vi "Drive_Motion_Control.vi"() -> ()   [LabVIEW 2017]
uses:
  State Control.ctl
panel:
  in  "Emergency Stop":bool
  out "Position":dbl(graph)
  out "Velocity":dbl(graph)
  in  "Move Absolute":bool
  in  "Move to Absolute Position in inches":dbl=1.0 min=1.0 max=20.0
  out "Motion in progress":bool
  in  "Homing":bool
  out "Sending in Progress":bool
  in  "Quit":bool
  in  "Motion Relative to Current Position (inch, + ext, - ret)":dbl
  out "Received Messages":string
  in  "Send command to MDrive":string
  out "Report":string
  in  "Parameters file":path=path "E:/thermionics/parameters.txt"
  in  "Move relative":bool
  in  "Send CTRL C":bool
  in  "Send command string":bool
  in  "Send parameters\nfrom file":bool
  # "Sendig file in progress"
  # "Motion in progress"
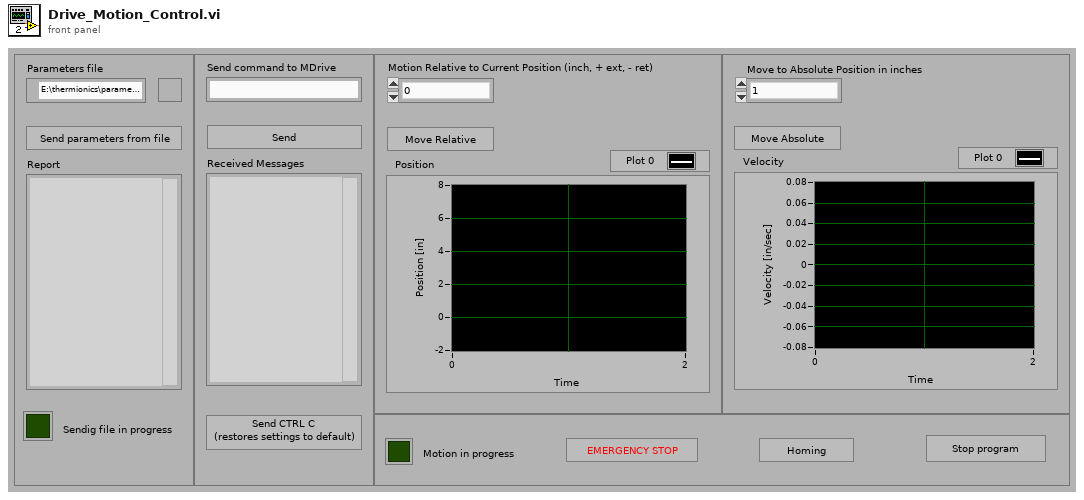
[diagram p1: front panel]
types:
  T1 = typedef "State Control.ctl" = enum16{"Check what pressed", "Send parameters file", "Send commad string", "Send ctrl c", "Move relative", "Move Absolute", "Homing", "Motion in progress", "Emergency stop"}
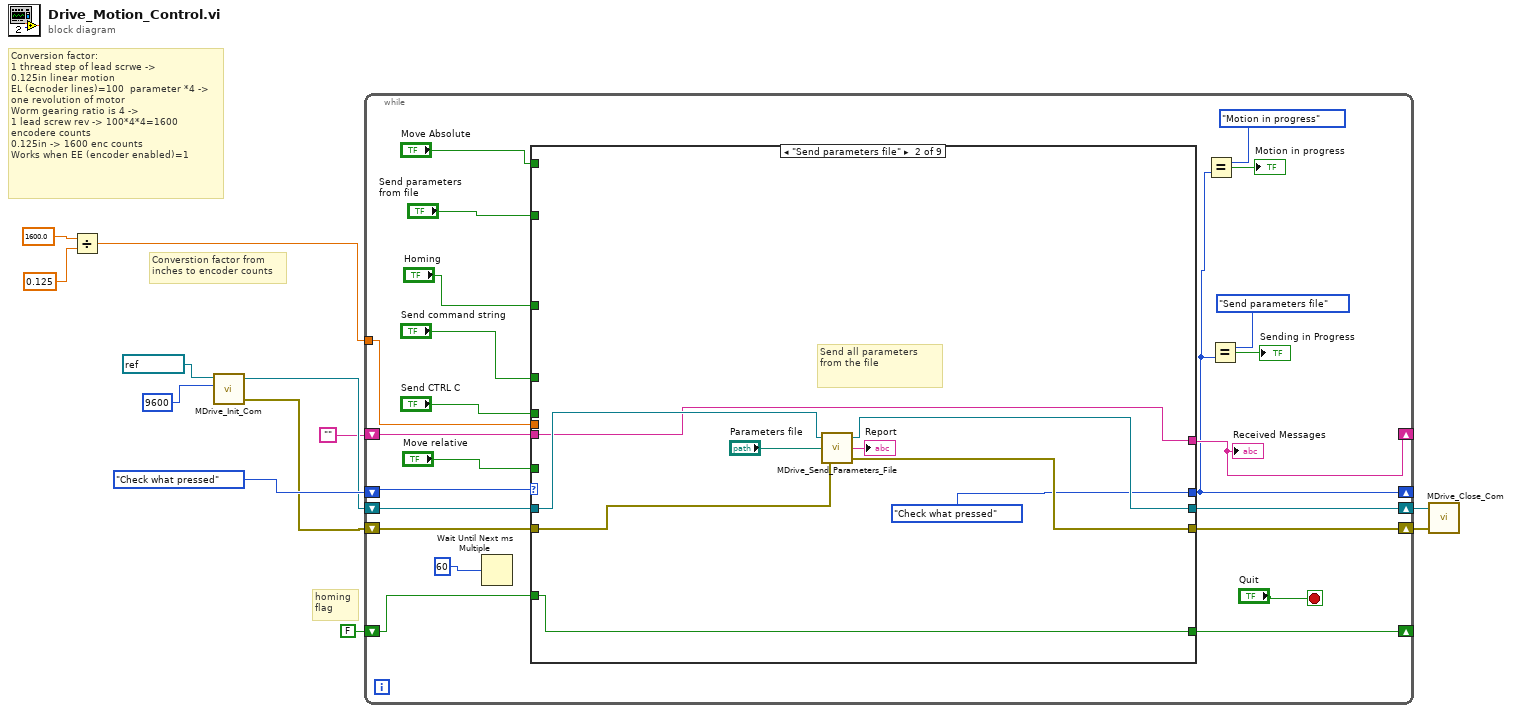
[diagram p0: block diagram]
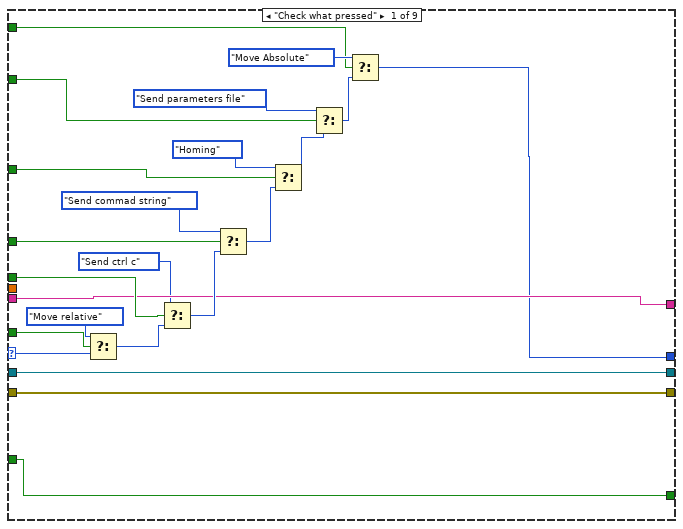
[diagram p2: hidden frame]
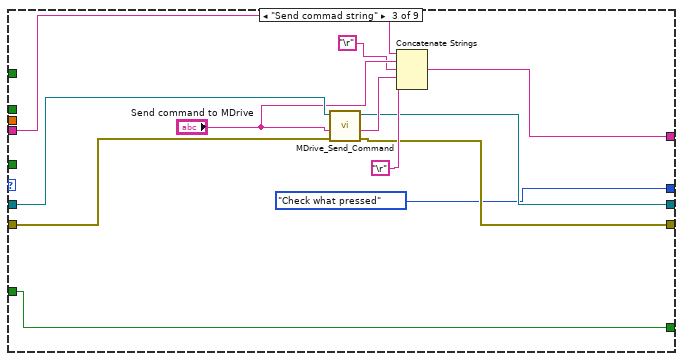
[diagram p3: hidden frame]
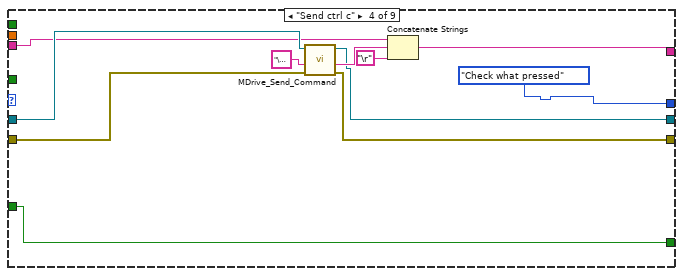
[diagram p4: hidden frame]
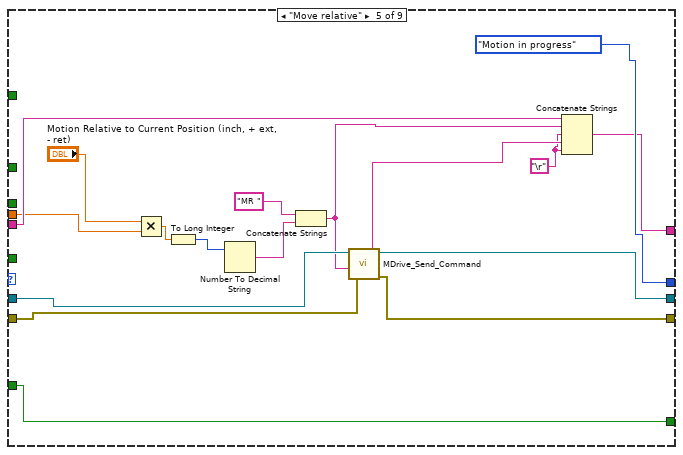
[diagram p5: hidden frame]
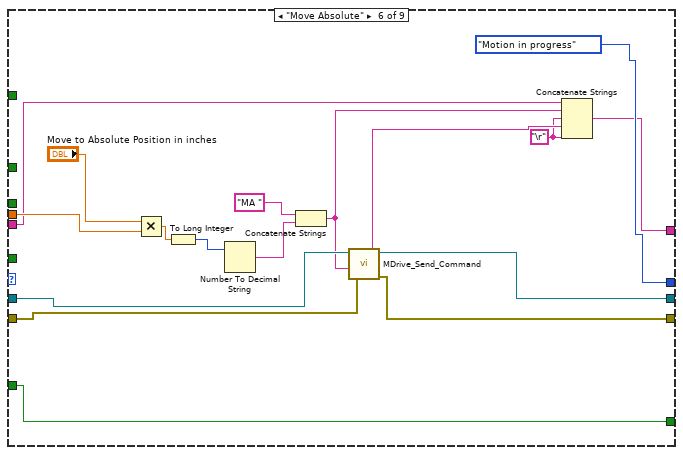
[diagram p6: hidden frame]
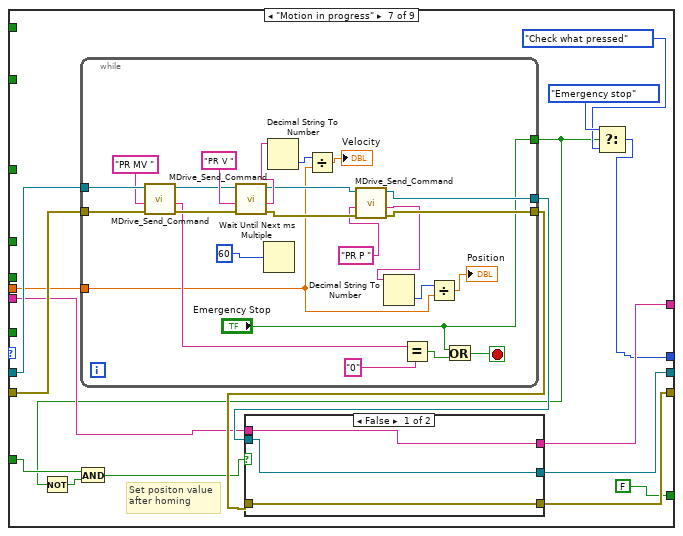
[diagram p7: hidden frame]
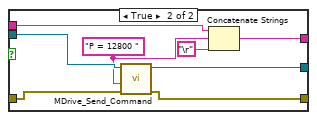
[diagram p8: hidden frame]
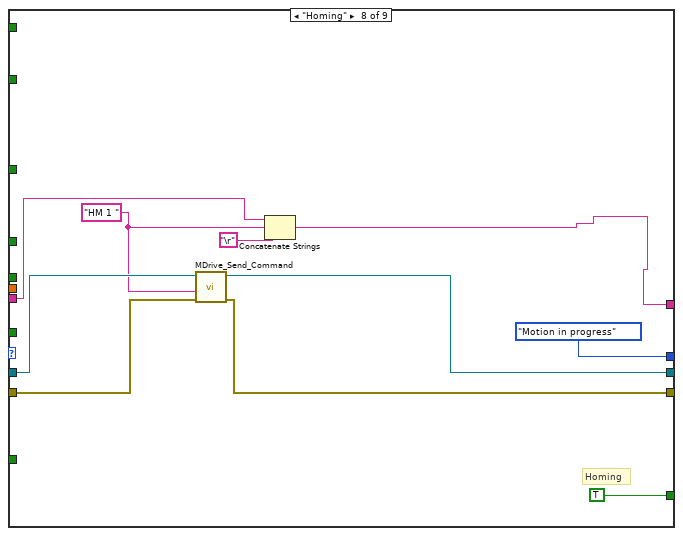
[diagram p9: hidden frame]
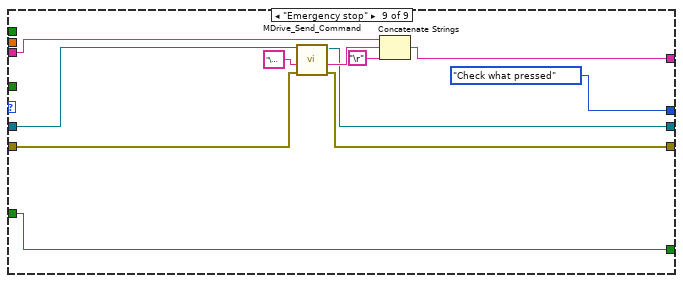
[diagram p10: hidden frame]
diagram:
  # "homing\nflag"
  # "Converstion factor from\ninches to encoder counts"
  # "Conversion factor:\n1 thread step of lead scrwe ->\n0.125in linear motion\nEL (ecnoder lines)=100  parameter *4 ->\none revolution of motor\nWorm gearing ratio is 4 ->\n1 lead screw rev -> 100*4*4=1600 encodere counts\n0.125in -> 1600 enc counts\nWorks when EE (encoder enabled)=1"
  n1 = Divide(x=1600.0 ("y"), y=0.125) -> (x/y=w2:dbl)
  n2 = call "MDrive_Init_Com.vi"("VISA resource name"=refnum<visa-resource-name> "COM4", "baud rate"=u32 9600) -> ("VISA resource name out"=w10:refnum<visa-resource-name>, "error out"=w11:errorcluster)  [unwired: 5 in]
  n3 = while {
    shift-right: [w34] -> w8
    shift-left: w10 -> [w32]
    shift-right: [w35] -> w9
    shift-left: w11 -> [w31]
    shift-right: [w15] -> _
    shift-left: State_Control."Check what pressed" ("Enum") -> [w30]
    shift-right: [w25] -> _
    shift-left: "" -> [w26]
    tunnel: w2 -> [w16]
    shift-right: [w14] -> _
    shift-left: FALSE -> [w13]
    stop <- "Quit" stop-if-true
    n4 = Wait Until Next ms Multiple(millisecond multiple=u32 60) -> ()  [unwired: 1 out]
    n5 = case shown="\"Send parameters file\"" w30 {
      selector: w30 -> [w55 _ _ _ _ _ _ _ _]
      tunnel: [w57 w62 w74 w86 w96 w113 w138 w179 w188] -> w35
      tunnel: [w58 w63 w75 w84 w95 w112 w136 w180 w187] -> w34
      tunnel: "Send parameters\nfrom file" -> [w56 _ _ _ _ _ _ _ _]
      tunnel: w32 -> [w58 w64 w77 w85 w103 w120 w140 w186 w192]
      tunnel: w31 -> [w57 w65 w76 w87 w102 w119 w141 w185 w193]
      tunnel: "Move relative" -> [w54 _ _ _ _ _ _ _ _]
      tunnel: "Send CTRL C" -> [w52 _ _ _ _ _ _ _ _]
      tunnel: "Send command string" -> [w50 _ _ _ _ _ _ _ _]
      tunnel: [w36 State_Control."Check what pressed" ("Enum") State_Control."Check what pressed" ("Enum") State_Control."Check what pressed" ("Enum") State_Control."Motion in progress" ("Enum") State_Control."Motion in progress" ("Enum") w130 State_Control."Motion in progress" ("Enum") State_Control."Check what pressed" ("Enum")] -> w15
      tunnel: [w49 w61 w73 w83 w99 w116 w132 w181 w190] -> w25
      tunnel: w26 -> [w49 w61 w70 w82 w100 w110 w133 w182 w191]
      tunnel: "Homing" -> [w46 _ _ _ _ _ _ _ _]
      tunnel: "Move Absolute" -> [w38 _ _ _ _ _ _ _ _]
      tunnel: w16 -> [_ _ _ _ w98 w114 w135 _ _]
      tunnel: [w37 w59 w71 w80 w94 w111 FALSE TRUE w197] -> w14
      tunnel: w13 -> [w37 w59 w71 w80 w94 w111 w127 _ w197]
      frame "Check what pressed" {
        n6 = Select(t=State_Control."Move relative", s=w54, f=w55) -> (s? t:f=w53:T1)
        n7 = Select(t=State_Control."Send ctrl c", s=w52, f=w53) -> (s? t:f=w51:T1)
        n8 = Select(t=State_Control."Send commad string", s=w50, f=w51) -> (s? t:f=w48:T1)
        n9 = Select(t=State_Control."Homing", s=w46, f=w48) -> (s? t:f=w47:T1)
        n10 = Select(t=State_Control."Send parameters file", s=w56, f=w47) -> (s? t:f=w40:T1)
        n11 = Select(t=State_Control."Move Absolute", s=w38, f=w40) -> (s? t:f=w36:T1)
      }
      frame "Send parameters file" {
        # "Send all parameters\nfrom the file"
        n12 = call "MDrive_Send_Parameters_File.vi"("error in"=w65, "parameters file"="Parameters file", "VISA resource name in"=w64) -> ("error in 2"=w62:errorcluster, "Report"=→"Report":string, "VISA resource name in 2"=w63:refnum<visa-resource-name>)
      }
      frame "Send commad string" {
        n13 = call "MDrive_Send_Command.vi"("error in"=w76, "Send String"="Send command to MDrive", "VISA resource name in"=w77) -> ("error out"=w74:errorcluster, "read buffer"=w79:string, "VISA resource name out"=w75:refnum<visa-resource-name>)  [unwired: 2 in]
        n14 = Concatenate Strings(w70, "Send command to MDrive", "\r", w79, "\r") -> (w73:string)
      }
      frame "Send ctrl c" {
        n15 = call "MDrive_Send_Command.vi"("error in"=w87, "Send String"="\u0003", "VISA resource name in"=w85) -> ("error out"=w86:errorcluster, "read buffer"=w90:string, "VISA resource name out"=w84:refnum<visa-resource-name>)  [unwired: 2 in]
        n16 = Concatenate Strings(w82, w90, "\r") -> (w83:string)
      }
      frame "Move relative" {
        w91 = "\r"
        n17 = Multiply(x="Motion Relative to Current Position (inch, + ext, - ret)", y=w98) -> (x*y=w105:dbl)
        n18 = To Long Integer(number=w105) -> (32bit integer=w106:i32)
        n19 = Number To Decimal String(number=w106) -> (decimal integer string=w107:string)  [unwired: 1 in]
        n20 = Concatenate Strings("MR ", w107) -> (w92:string)
        n21 = call "MDrive_Send_Command.vi"("error in"=w102, "Send String"=w92, "VISA resource name in"=w103) -> ("error out"=w96:errorcluster, "read buffer"=w93:string, "VISA resource name out"=w95:refnum<visa-resource-name>)  [unwired: 2 in]
        n22 = Concatenate Strings(w100, w92, w91, w93, w91) -> (w99:string)
      }
      frame "Move Absolute" {
        w108 = "\r"
        n23 = Multiply(x="Move to Absolute Position in inches", y=w114) -> (x*y=w122:dbl)
        n24 = To Long Integer(number=w122) -> (32bit integer=w123:i32)
        n25 = Number To Decimal String(number=w123) -> (decimal integer string=w124:string)  [unwired: 1 in]
        n26 = Concatenate Strings("MA ", w124) -> (w109:string)
        n27 = call "MDrive_Send_Command.vi"("error in"=w119, "Send String"=w109, "VISA resource name in"=w120) -> ("error out"=w113:errorcluster, "read buffer"=w117:string, "VISA resource name out"=w112:refnum<visa-resource-name>)  [unwired: 2 in]
        n28 = Concatenate Strings(w110, w109, w108, w117, w108) -> (w116:string)
      }
      frame "Motion in progress" {
        # "Set positon value\nafter homing"
        n29 = while {
          tunnel: [w163] -> w139
          tunnel: [w162] -> w137
          tunnel: w141 -> [w169]
          tunnel: w140 -> [w168]
          tunnel: w135 -> [w158]
          tunnel: ["Emergency Stop"] -> w126
          stop <- w154 stop-if-true
          n30 = call "MDrive_Send_Command.vi"("error in"=w169, "Send String"="PR MV ", "VISA resource name in"=w168) -> ("error out"=w171:errorcluster, "read buffer"=w166:string, "VISA resource name out"=w170:refnum<visa-resource-name>)  [unwired: 2 in]
          n31 = call "MDrive_Send_Command.vi"("error in"=w171, "Send String"="PR V ", "VISA resource name in"=w170) -> ("error out"=w164:errorcluster, "read buffer"=w174:string, "VISA resource name out"=w161:refnum<visa-resource-name>)  [unwired: 2 in]
          n32 = Wait Until Next ms Multiple(millisecond multiple=u32 60) -> ()  [unwired: 1 out]
          n33 = Decimal String To Number(string=w174) -> (number=w172:i32)  [unwired: 2 in, 1 out]
          n34 = Divide(x=w172, y=w158) -> (x/y=→"Velocity":dbl)
          n35 = call "MDrive_Send_Command.vi"("error in"=w164, "Send String"="PR P ", "VISA resource name in"=w161) -> ("error out"=w163:errorcluster, "read buffer"=w156:string, "VISA resource name out"=w162:refnum<visa-resource-name>)  [unwired: 2 in]
          n36 = Decimal String To Number(string=w156) -> (number=w159:i32)  [unwired: 2 in, 1 out]
          n37 = Equal?(x=w166, y="0") -> (x = y?=w155:bool)
          n38 = Divide(x=w159, y=w158) -> (x/y=→"Position":dbl)
          n39 = Or(x="Emergency Stop", y=w155) -> (x .or. y?=w154:bool)
        }
        n40 = Not(x=w126) -> (.not. x?=w125:bool)
        n41 = And(x=w127, y=w125) -> (x .and. y?=w128:bool)
        n42 = case shown="False" w128 {
          tunnel: w139 -> [w144 w152]
          tunnel: [w144 w151] -> w138
          tunnel: w137 -> [w143 w150]
          tunnel: [w143 w149] -> w136
          tunnel: w133 -> [w142 w147]
          tunnel: [w142 w146] -> w132
          frame False {
          }
          frame True {
            w145 = "P = 12800 "
            n43 = call "MDrive_Send_Command.vi"("error in"=w152, "Send String"=w145, "VISA resource name in"=w150) -> ("error out"=w151:errorcluster, "VISA resource name out"=w149:refnum<visa-resource-name>)  [unwired: 2 in, 1 out]
            n44 = Concatenate Strings(w147, w145, "\r") -> (w146:string)
          }
        }
        n45 = Select(t=State_Control."Emergency stop", s=w126, f=State_Control."Check what pressed" ("Enum")) -> (s? t:f=w130:T1)
      }
      frame "Homing" {
        w177 = "HM 1 "
        # "Homing"
        n46 = call "MDrive_Send_Command.vi"("error in"=w185, "Send String"=w177, "VISA resource name in"=w186) -> ("error out"=w179:errorcluster, "VISA resource name out"=w180:refnum<visa-resource-name>)  [unwired: 2 in, 1 out]
        n47 = Concatenate Strings(w182, w177, "\r") -> (w181:string)
      }
      frame "Emergency stop" {
        n48 = call "MDrive_Send_Command.vi"("error in"=w193, "Send String"="\u001b", "VISA resource name in"=w192) -> ("error out"=w188:errorcluster, "read buffer"=w196:string, "VISA resource name out"=w187:refnum<visa-resource-name>)  [unwired: 2 in]
        n49 = Concatenate Strings(w191, w196, "\r") -> (w190:string)
      }
    }
    "Received Messages" <- w25
    n50 = Equal?(x=State_Control."Motion in progress", y=w15) -> (x = y?=→"Motion in progress":bool)
    n51 = Equal?(x=State_Control."Send parameters file", y=w15) -> (x = y?=→"Sending in Progress":bool)
  }
  n52 = call "MDrive_Close_Com.vi"("error out"=w9, "VISA resource name out"=w8) -> ()  [unwired: 2 in]
